vi "pratik1 (SubVI).vi"(1 "Input String":string) -> (0 "Cluster":T1={"Ch1 Voltage Digit Color"={"White"=FALSE, "Green "=FALSE, "Gray"=FALSE, "Magenta"=FALSE, "default"=TRUE}, "Ch1 Frame Color"={"Green"=FALSE, "Gray"=FALSE, "Yellow"=FALSE, "White"=FALSE, "default"=TRUE}, "Ch1 Outflow Tube"={"White"=FALSE, "Green"=FALSE, "Gray"=FALSE, "default"=TRUE}, "Ch1 Current Digit Color "={"White"=FALSE, "Green"=FALSE, "Gray"=FALSE, "Magenta"=FALSE, "default"=TRUE}})   [LabVIEW 2024]
panel:
  out "Byte 1":dbl
  out "Byte 0":dbl
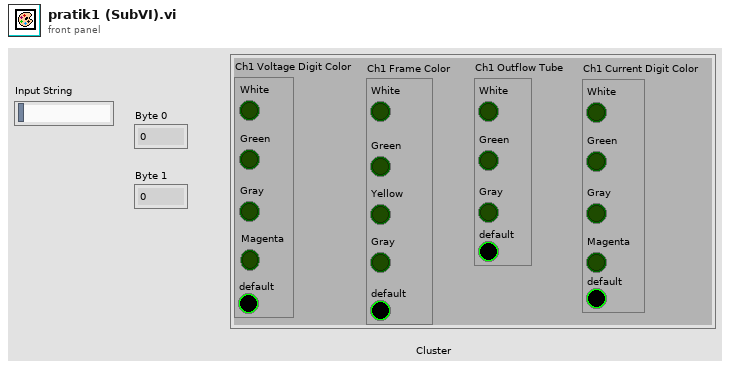
[diagram p1: front panel]
types:
  T1 = cluster{"Ch1 Voltage Digit Color":cluster{"White":bool, "Green ":bool, "Gray":bool, "Magenta":bool, "default":bool}, "Ch1 Frame Color":cluster{"Green":bool, "Gray":bool, "Yellow":bool, "White":bool, "default":bool}, "Ch1 Outflow Tube":cluster{"White":bool, "Green":bool, "Gray":bool, "default":bool}, "Ch1 Current Digit Color ":cluster{"White":bool, "Green":bool, "Gray":bool, "Magenta":bool, "default":bool}}
  T2 = cluster{"White":bool, "Green":bool, "Gray 4":bool, "Magenta 4":bool, "default 3":bool}
  T3 = cluster{"White":bool, "Green":bool, "Gray 3":bool, "default 2":bool}
  T4 = cluster{"Green":bool, "Gray":bool, "Yellow":bool, "White":bool, "default":bool}
  T5 = cluster{"White":bool, "Green ":bool, "Gray":bool, "Magenta":bool, "default":bool}
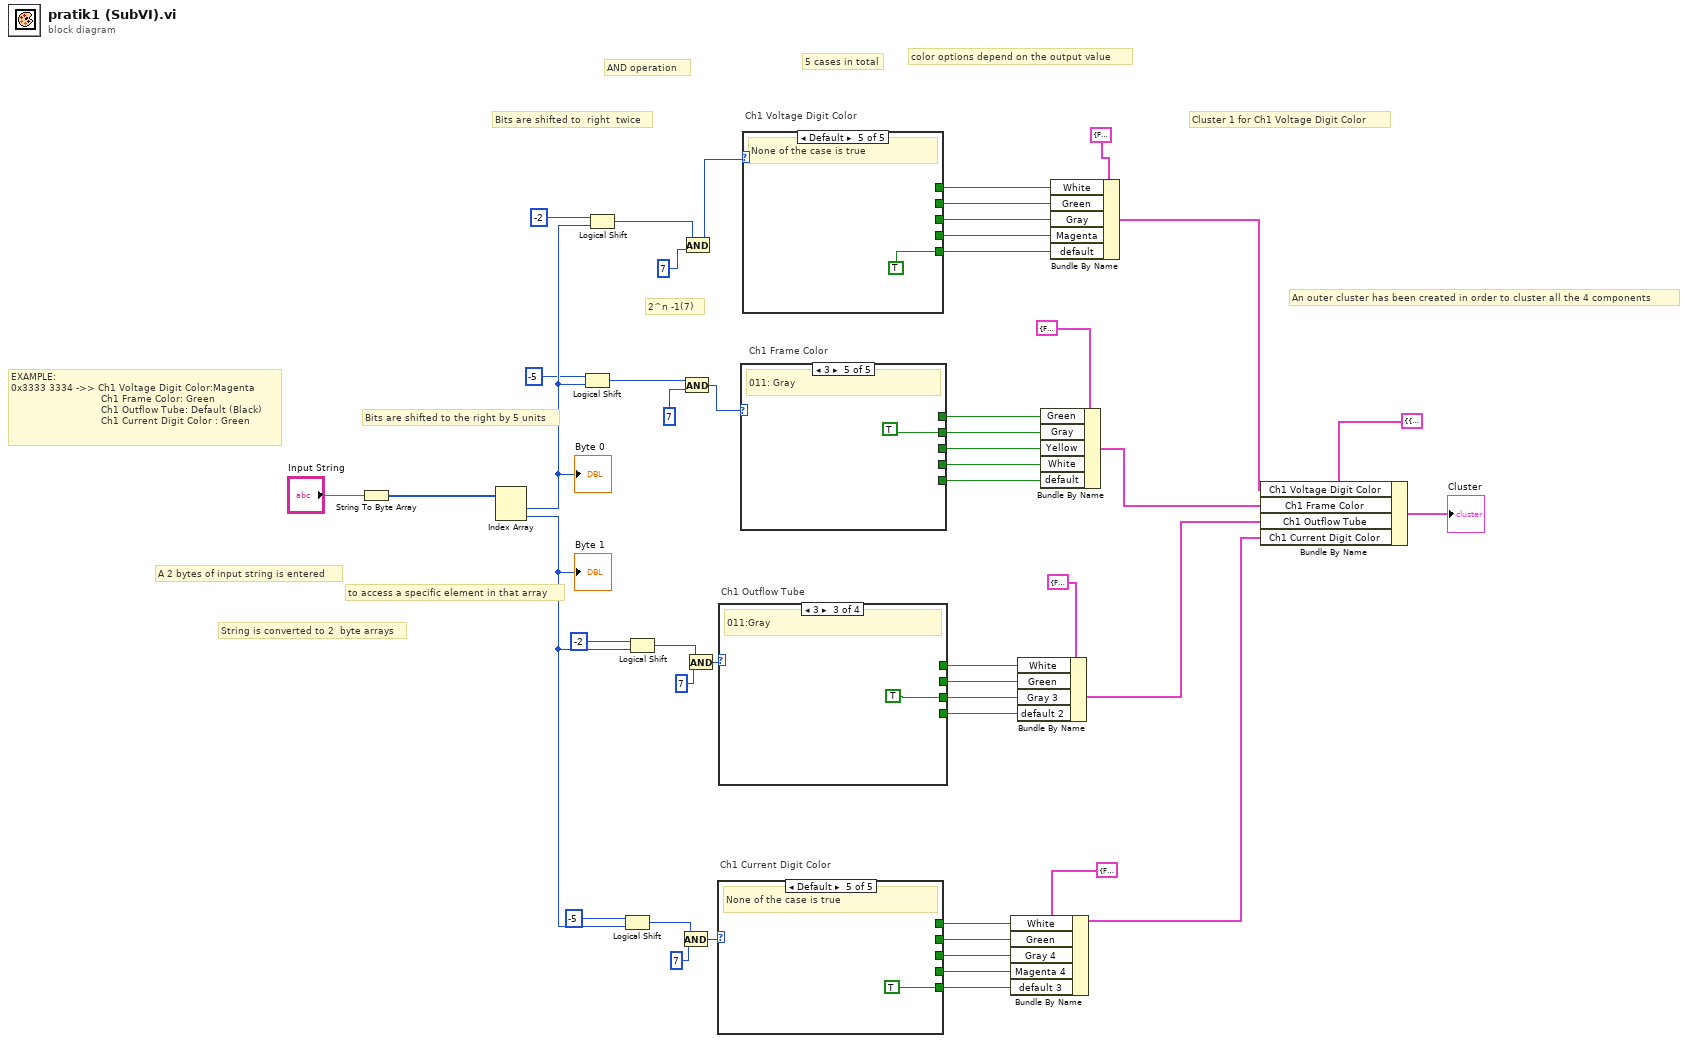
[diagram p0: block diagram]
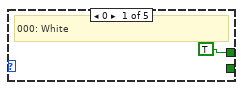
[diagram p2: hidden frame]
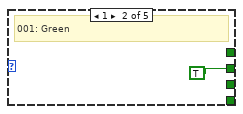
[diagram p3: hidden frame]
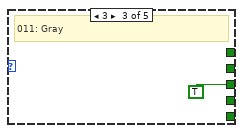
[diagram p4: hidden frame]
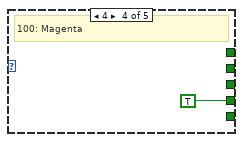
[diagram p5: hidden frame]
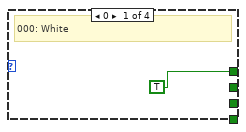
[diagram p6: hidden frame]
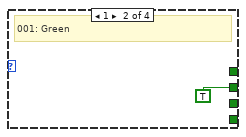
[diagram p7: hidden frame]
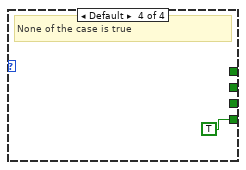
[diagram p8: hidden frame]
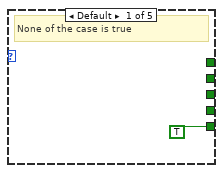
[diagram p9: hidden frame]
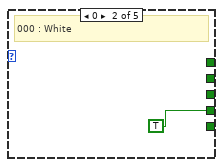
[diagram p10: hidden frame]
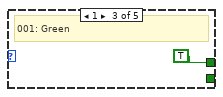
[diagram p11: hidden frame]
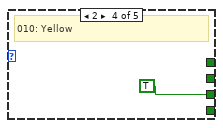
[diagram p12: hidden frame]
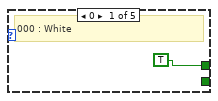
[diagram p13: hidden frame]
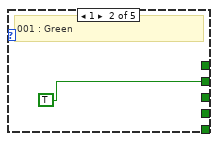
[diagram p14: hidden frame]
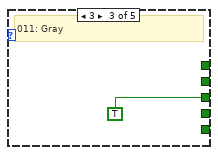
[diagram p15: hidden frame]
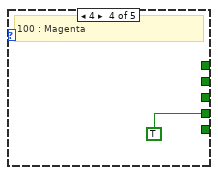
[diagram p16: hidden frame]
diagram:
  # "EXAMPLE: \n0x3333 3334 ->> Ch1 Voltage Digit Color:Magenta\n                              Ch1 Frame Color: Green\n                              Ch1 Outflow Tube: Default (Black)\n                              Ch1 Current Digit Color : Green"
  # "5 cases in total"
  # "color options depend on the output value"
  # "Cluster 1 for Ch1 Voltage Digit Color"
  # "Bits are shifted to the right by 5 units"
  # "2^n -1(7)"
  # "AND operation"
  # "Bits are shifted to  right  twice"
  # "to access a specific element in that array"
  # "String is converted to 2  byte arrays"
  # "A 2 bytes of input string is entered"
  # "An outer cluster has been created in order to cluster all the 4 components"
  # "Ch1 Current Digit Color"
  # "Ch1 Outflow Tube"
  # "Ch1 Frame Color"
  # "Ch1 Voltage Digit Color"
  n1 = String To Byte Array(string="Input String") -> (unsigned byte array=w48:u8[])
  n2 = Index Array "Index Array"(array=w48) -> (element #1=w43:u8, element #2=w30:u8)  [unwired: 2 in]
  "Byte 0" <- w43
  "Byte 1" <- w30
  n3 = Logical Shift(y=i16 -5, x=w43) -> (x << y=w41:u8)
  n4 = Logical Shift(y=i16 -2, x=w43) -> (x << y=w46:u8)
  n5 = Logical Shift(y=i16 -5, x=w30) -> (x << y=w33:u8)
  n6 = Logical Shift(y=i16 -2, x=w30) -> (x << y=w37:u8)
  n7 = And(x=w33, y=u8 7) -> (x .and. y?=w31:u8)
  n8 = And(x=w41, y=u8 7) -> (x .and. y?=w39:u8)
  n9 = And(x=w46, y=u8 7) -> (x .and. y?=w44:u8)
  n10 = And(x=w37, y=u8 7) -> (x .and. y?=w35:u8)
  n11 = case shown="Default" w31 {
    tunnel: [_ _ _ _ TRUE ("default 3")] -> w16
    tunnel: [TRUE ("White 4") _ _ _ _] -> w15
    tunnel: [_ TRUE ("Green  2") _ _ _] -> w14
    tunnel: [_ _ TRUE ("Gray 4") _ _] -> w13
    tunnel: [_ _ _ TRUE ("Magenta 4") _] -> w12
    frame 0 {
      # "000: White"
    }
    frame 1 {
      # "001: Green"
    }
    frame 3 {
      # "011: Gray"
    }
    frame 4 {
      # "100: Magenta"
    }
    frame Default {
      # "None of the case is true"
    }
  }
  n12 = case shown="3" w35 {
    tunnel: [TRUE ("White 3") _ _ _] -> w21
    tunnel: [_ TRUE ("Green  2") _ _] -> w20
    tunnel: [_ _ TRUE ("Gray 3") _] -> w19
    tunnel: [_ _ _ TRUE ("default 2")] -> w18
    frame 0 {
      # "000: White"
    }
    frame 1 {
      # "001: Green"
    }
    frame 3 {
      # "011:Gray"
    }
    frame Default {
      # "None of the case is true"
    }
  }
  n13 = case shown="3" w39 {
    tunnel: [_ TRUE ("White 2") _ _ _] -> w5
    tunnel: [_ _ TRUE ("Green  2") _ _] -> w4
    tunnel: [_ _ _ TRUE ("Gray") _] -> w3
    tunnel: [_ _ _ _ TRUE ("Yellow")] -> w2
    tunnel: [TRUE ("default 2") _ _ _ _] -> w1
    frame Default {
      # "None of the case is true"
    }
    frame 0 {
      # "000 : White"
    }
    frame 1 {
      # "001: Green"
    }
    frame 2 {
      # "010: Yellow"
    }
    frame 3 {
      # "011: Gray"
    }
  }
  n14 = case shown="Default" w44 {
    tunnel: [TRUE ("Boolean") _ _ _ _] -> w28
    tunnel: [_ TRUE ("Boolean 2") _ _ _] -> w27
    tunnel: [_ _ TRUE ("Boolean 3") _ _] -> w26
    tunnel: [_ _ _ TRUE ("Boolean 4") _] -> w25
    tunnel: [_ _ _ _ TRUE ("defalt")] -> w24
    frame 0 {
      # "000 : White"
    }
    frame 1 {
      # "001 : Green"
    }
    frame 3 {
      # "011: Gray"
    }
    frame 4 {
      # "100 : Magenta"
    }
    frame Default {
      # "None of the case is true"
    }
  }
  n15 = Bundle By Name(cluster=T2 {"White"=FALSE, "Green"=FALSE, "Gray 4"=FALSE, "Magenta 4"=FALSE, "default 3"=FALSE} ("Ch1 Current Digit Color"), "White"=w15, "Green"=w14, "Gray 4"=w13, "Magenta 4"=w12, "default 3"=w16) -> (w6:T2)
  n16 = Bundle By Name(cluster=T3 {"White"=FALSE, "Green"=FALSE, "Gray 3"=FALSE, "default 2"=FALSE} ("Ch1 Outflow Tube"), "White"=w21, "Green"=w20, "Gray 3"=w19, "default 2"=w18) -> (w7:T3)
  n17 = Bundle By Name(cluster=T4 {"Green"=FALSE, "Gray"=FALSE, "Yellow"=FALSE, "White"=FALSE, "default"=FALSE} ("Ch1 Frame Color"), "Green"=w4, "Gray"=w2, "Yellow"=w3, "White"=w5, "default"=w1) -> (w8:T4)
  n18 = Bundle By Name(cluster=T5 {"White"=FALSE, "Green "=FALSE, "Gray"=FALSE, "Magenta"=FALSE, "default"=FALSE} ("Voltage Digit"), "White"=w28, "Green"=w27, "Gray"=w26, "Magenta"=w25, "default"=w24) -> (w9:T5)
  n19 = Bundle By Name(cluster=T1 {"Ch1 Voltage Digit Color"={"White"=FALSE, "Green "=FALSE, "Gray"=FALSE, "Magenta"=FALSE, "default"=FALSE}, "Ch1 Frame Color"={"Green"=FALSE, "Gray"=FALSE, "Yellow"=FALSE, "White"=FALSE, "default"=FALSE}, "Ch1 Outflow Tube"={"White"=FALSE, "Green"=FALSE, "Gray"=FALSE, "default"=FALSE}, "Ch1 Current Digit Color "={"White"=FALSE, "Green"=FALSE, "Gray"=FALSE, "Magenta"=FALSE, "default"=FALSE}} ("Cluster"), "Ch1 Voltage Digit Color"=w9, "Ch1 Frame Color"=w8, "Ch1 Outflow Tube"=w7, "Ch1 Current Digit Color"=w6) -> (→"Cluster":T1)
